vi "ErrorHandlerModularLoop vxm.vi"(8 "error in (no error)":errorcluster, 9 "exit event source":refnum<user-event>, 11 "MessageQues":T1) -> (0 "error out":errorcluster)   [LabVIEW 2019]
doc: "The Error hanlder Loop handles errors from all other Loops in the Multiple Loop Application Framework.\n\nThe DAQ Loop might need special handling, placeholde only now.\n\nMain and Analysis are set up to just Flush their ques, clear the error and pop open an OK dialog.\n***Not sure how we'll handle an error where messages are continually dropped on the Analysis/Main Que, causing the same error to repeat over and over - handle when needed."
uses:
  MessageQue/VXM Main Test App/MultipleMessageQues vxm.ctl
  MessageQue/MessageQue.ctl
  MessageQue/MessageCluster.ctl
  <vilib>/Utility/error.llb/DialogTypeEnum.ctl
  MessageQue/MessageQue.lvlib
  UserEvent-ExitEventLoop/UserEvent-ExitEventLoop.lvlib
panel:
  out "i":i32
  out "Command":string
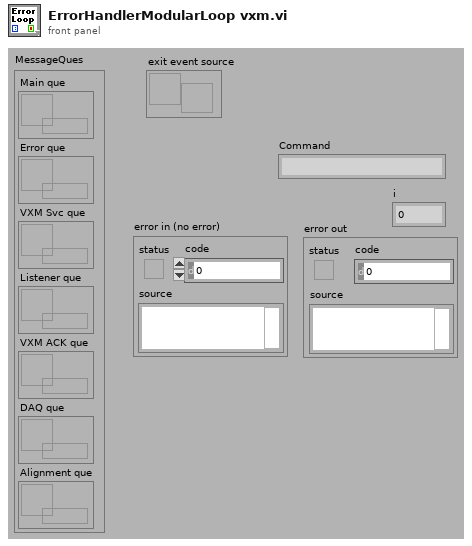
[diagram p1: front panel]
types:
  T1 = typedef "MultipleMessageQues vxm.ctl" = cluster{"Main que":T2, "Error que":T2, "VXM Svc que":T2, "Listener que":T2, "VXM ACK que":T2, "DAQ que":T2, "Alignment que":T2}
  T2 = typedef "MessageQue.lvlib/MessageQue.ctl" = refnum<queue>
  T3 = typedef "DialogTypeEnum.ctl" = enum16{"no dialog", "OK message", "continue or stop message", "auto error handling dialog", "OK message + warnings", "continue/stop + warnings"}
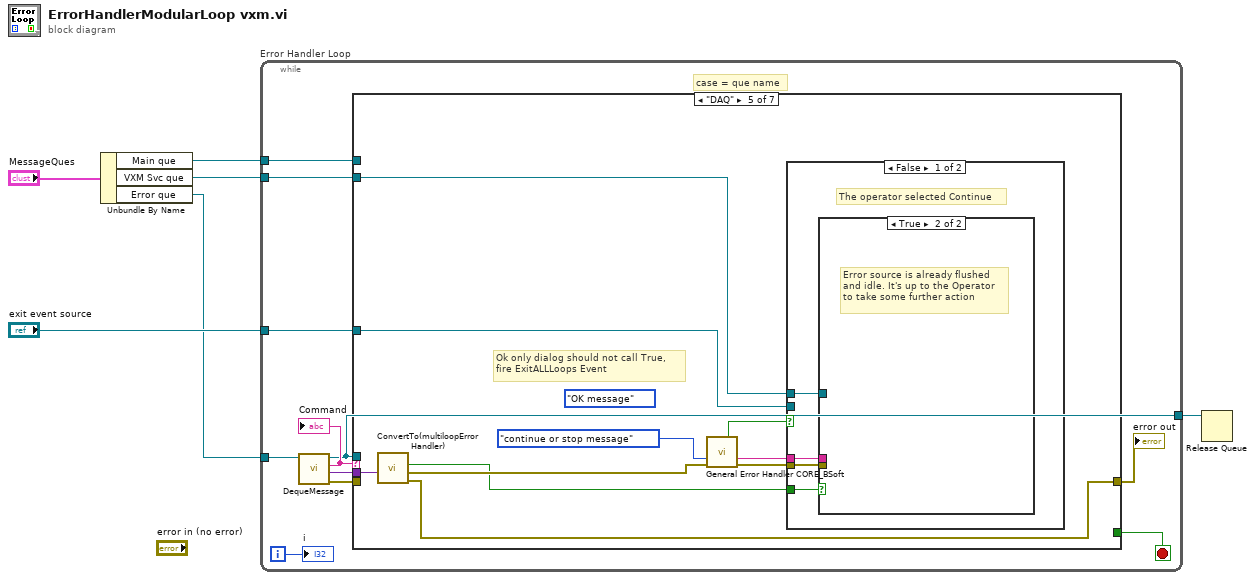
[diagram p0: block diagram]
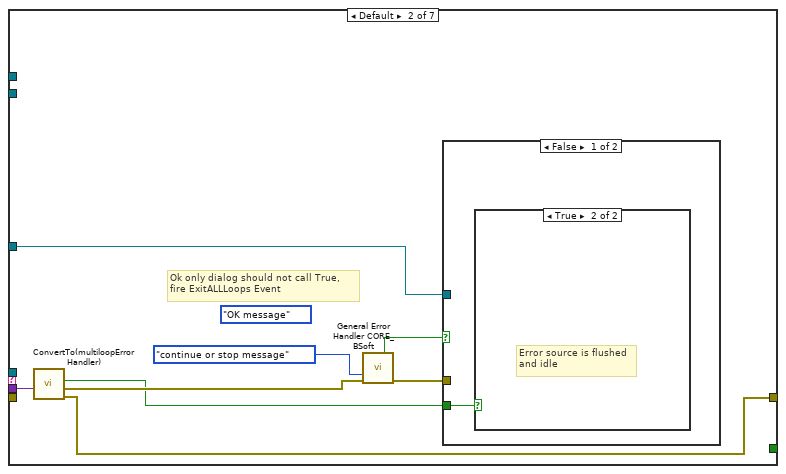
[diagram p3: hidden frame]
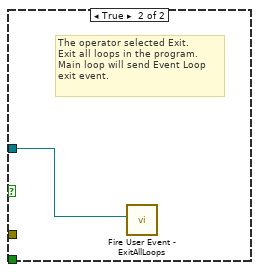
[diagram p5: hidden frame]
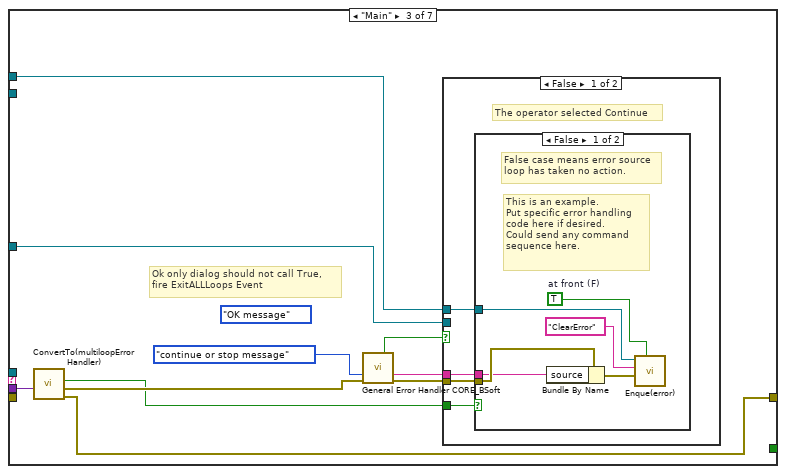
[diagram p6: hidden frame]
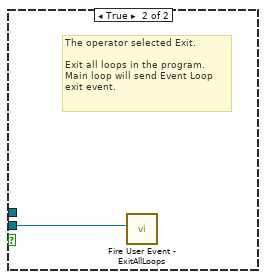
[diagram p8: hidden frame]
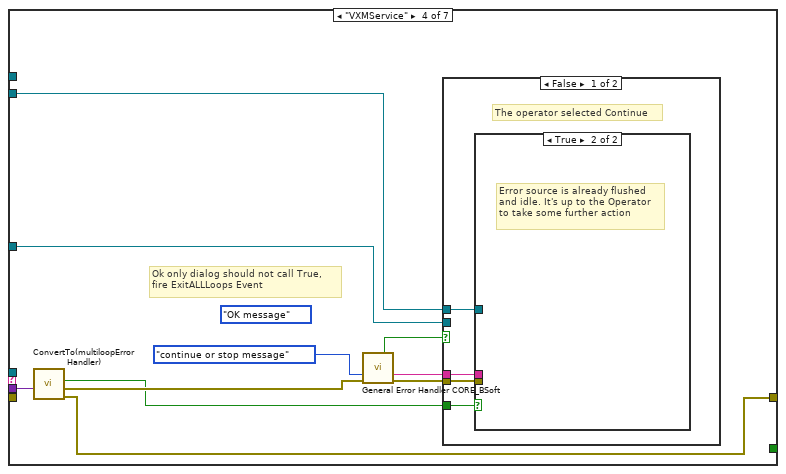
[diagram p9: hidden frame]
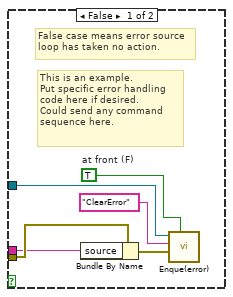
[diagram p10: hidden frame]
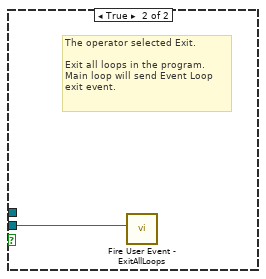
[diagram p11: hidden frame]
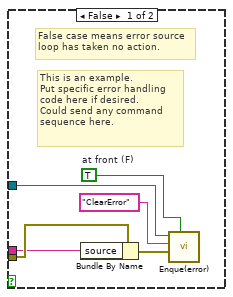
[diagram p12: hidden frame]
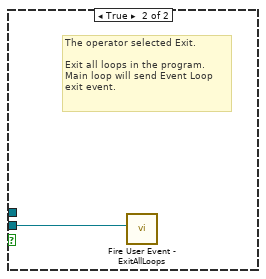
[diagram p13: hidden frame]
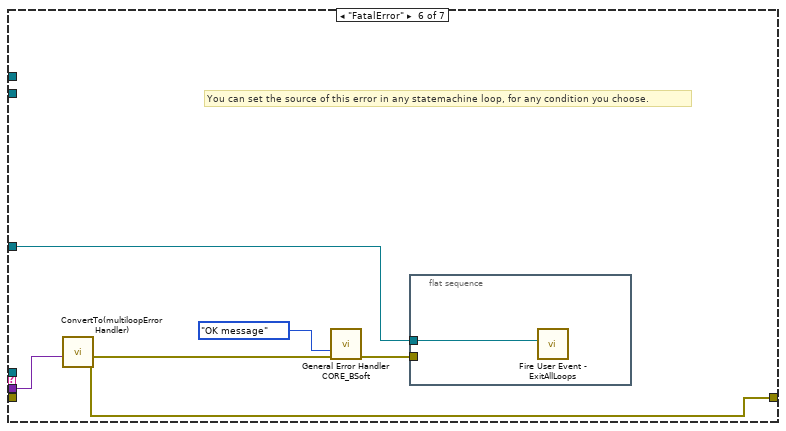
[diagram p14: hidden frame]
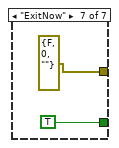
[diagram p15: hidden frame]
diagram:
  n1 = Unbundle By Name("MessageQues") -> ("Main que"=w3:T2, "VXM Svc que"=w4:T2, "Error que"=w2:T2)
  n2 = while "Error Handler Loop" {
    tunnel: w2 -> [w17]
    tunnel: w3 -> [w12]
    tunnel: w4 -> [w11]
    tunnel: "exit event source" -> [w9]
    tunnel: [w8] -> w5
    i -> [w16]
    stop <- w13 stop-if-true
    # "case = que name"
    n3 = call "DequeMessage.vi"("Message que"=w17) -> ("error out"=w14:errorcluster, "Message Payload"=w7:variant, "Message Command"=w15:string, "Message que out"=w8:T2)  [unwired: 5 in, 2 out]
    "Command" <- w15
    n4 = case shown="\"DAQ\"" w15 {
      tunnel: w8 -> [_ _ _ _ _ _ _]
      tunnel: [w18 w25 w37 w58 w79 w96 errorcluster {"status"=FALSE, "code"=0, "source"=""} ("error in (no error)")] -> w10
      tunnel: w14 -> [w18 _ _ _ _ _ _]
      tunnel: [_ _ _ _ _ _ TRUE] -> w13
      tunnel: w7 -> [_ w24 w36 w57 w78 w97 _]
      tunnel: w12 -> [_ _ w29 _ _ _ _]
      tunnel: w11 -> [_ _ _ w50 w71 _ _]
      tunnel: w9 -> [_ w26 w38 w59 w80 w92 _]
      frame "idle" {
      }
      frame Default {
        (unwired) DialogTypeEnum."OK message" ("type of dialog (OK msg:1)")
        # "Ok only dialog should not call True,\nfire ExitALLLoops Event"
        n5 = call "ConvertTo(multiloopErrorHandler).vi"("Message Payload"=w24) -> ("error out"=w25:errorcluster, "Message Payload error"=w20:errorcluster, "Handle Loop Que"=w19:bool)  [unwired: 8 in]
        n6 = call "General Error Handler CORE_BSoft.vi"("type of dialog (OK msg:1)"=DialogTypeEnum."continue or stop message", "error in (no error)"=w20) -> ("stop event propagated"=w23:bool, "error out"=w21:errorcluster)  [unwired: 8 in, 4 out]
        n7 = case shown="False" w23 {
          tunnel: w26 -> [_ w28]
          tunnel: w21 -> [_ _]
          tunnel: w19 -> [w27 _]
          frame False {
            n8 = case shown="True" w27 {
              frame False {
                # "False case means error source\nloop has taken no action."
                # "Default case can't send anything\nback to the source loop becasue\nit is the default and doesn't know\nwhich loop it is"
              }
              frame True {
                # "Error source is flushed\nand idle"
              }
            }
          }
          frame True {
            # "The operator selected Exit.\nExit all loops in the program.\nMain loop will send Event Loop\nexit event."
            n9 = call "Fire User Event - ExitAllLoops.vi"("user event ExitEventLoop"=w28) -> ()  [unwired: 10 in, 1 out]
          }
        }
      }
      frame "Main" {
        (unwired) DialogTypeEnum."OK message" ("type of dialog (OK msg:1)")
        # "Ok only dialog should not call True,\nfire ExitALLLoops Event"
        n10 = call "ConvertTo(multiloopErrorHandler).vi"("Message Payload"=w36) -> ("error out"=w37:errorcluster, "Message Payload error"=w32:errorcluster, "Handle Loop Que"=w31:bool)  [unwired: 8 in]
        n11 = call "General Error Handler CORE_BSoft.vi"("type of dialog (OK msg:1)"=DialogTypeEnum."continue or stop message", "error in (no error)"=w32) -> ("stop event propagated"=w35:bool, "message"=w30:string, "error out"=w33:errorcluster)  [unwired: 8 in, 3 out]
        n12 = case shown="False" w35 {
          tunnel: w38 -> [_ w49]
          tunnel: w33 -> [w41 _]
          tunnel: w31 -> [w42 _]
          tunnel: w30 -> [w40 _]
          tunnel: w29 -> [w39 _]
          frame False {
            # "The operator selected Continue"
            n13 = case shown="False" w42 {
              tunnel: w41 -> [w45 _]
              tunnel: w40 -> [w44 _]
              tunnel: w39 -> [w43 _]
              frame False {
                w46 = TRUE  # at front (F)
                # "False case means error source\nloop has taken no action."
                # "This is an example.\nPut specific error handling \ncode here if desired.\nCould send any command\nsequence here."
                n14 = Bundle By Name(cluster=w45, "source"=w44) -> (w47:errorcluster)
                n15 = call "Enque(error).vi"("at front (F)"=w46, "Message Payload  error cluster"=w47, "Message Command"="ClearError", "Message que"=w43) -> ()  [unwired: 6 in, 2 out]
              }
              frame True {
                # "Error source is already flushed\nand idle. It's up to the Operator\nto take some further action"
              }
            }
          }
          frame True {
            # "The operator selected Exit.\n\nExit all loops in the program.\nMain loop will send Event Loop\nexit event."
            n16 = call "Fire User Event - ExitAllLoops.vi"("user event ExitEventLoop"=w49) -> ()  [unwired: 10 in, 1 out]
          }
        }
      }
      frame "VXMService" {
        (unwired) DialogTypeEnum."OK message" ("type of dialog (OK msg:1)")
        # "Ok only dialog should not call True,\nfire ExitALLLoops Event"
        n17 = call "ConvertTo(multiloopErrorHandler).vi"("Message Payload"=w57) -> ("error out"=w58:errorcluster, "Message Payload error"=w53:errorcluster, "Handle Loop Que"=w52:bool)  [unwired: 8 in]
        n18 = call "General Error Handler CORE_BSoft.vi"("type of dialog (OK msg:1)"=DialogTypeEnum."continue or stop message", "error in (no error)"=w53) -> ("stop event propagated"=w56:bool, "message"=w51:string, "error out"=w54:errorcluster)  [unwired: 8 in, 3 out]
        n19 = case shown="False" w56 {
          tunnel: w59 -> [_ w70]
          tunnel: w54 -> [w62 _]
          tunnel: w52 -> [w63 _]
          tunnel: w51 -> [w61 _]
          tunnel: w50 -> [w60 _]
          frame False {
            # "The operator selected Continue"
            n20 = case shown="True" w63 {
              tunnel: w62 -> [w66 _]
              tunnel: w61 -> [w65 _]
              tunnel: w60 -> [w64 _]
              frame False {
                w67 = TRUE  # at front (F)
                # "False case means error source\nloop has taken no action."
                # "This is an example.\nPut specific error handling \ncode here if desired.\nCould send any command\nsequence here."
                n21 = Bundle By Name(cluster=w66, "source"=w65) -> (w68:errorcluster)
                n22 = call "Enque(error).vi"("at front (F)"=w67, "Message Payload  error cluster"=w68, "Message Command"="ClearError", "Message que"=w64) -> ()  [unwired: 6 in, 2 out]
              }
              frame True {
                # "Error source is already flushed\nand idle. It's up to the Operator\nto take some further action"
              }
            }
          }
          frame True {
            # "The operator selected Exit.\n\nExit all loops in the program.\nMain loop will send Event Loop\nexit event."
            n23 = call "Fire User Event - ExitAllLoops.vi"("user event ExitEventLoop"=w70) -> ()  [unwired: 10 in, 1 out]
          }
        }
      }
      frame "DAQ" {
        (unwired) DialogTypeEnum."OK message" ("type of dialog (OK msg:1)")
        # "Ok only dialog should not call True,\nfire ExitALLLoops Event"
        n24 = call "ConvertTo(multiloopErrorHandler).vi"("Message Payload"=w78) -> ("error out"=w79:errorcluster, "Message Payload error"=w74:errorcluster, "Handle Loop Que"=w73:bool)  [unwired: 8 in]
        n25 = call "General Error Handler CORE_BSoft.vi"("type of dialog (OK msg:1)"=DialogTypeEnum."continue or stop message", "error in (no error)"=w74) -> ("stop event propagated"=w77:bool, "message"=w72:string, "error out"=w75:errorcluster)  [unwired: 8 in, 3 out]
        n26 = case shown="False" w77 {
          tunnel: w80 -> [_ w91]
          tunnel: w75 -> [w83 _]
          tunnel: w73 -> [w84 _]
          tunnel: w72 -> [w82 _]
          tunnel: w71 -> [w81 _]
          frame False {
            # "The operator selected Continue"
            n27 = case shown="True" w84 {
              tunnel: w83 -> [w87 _]
              tunnel: w82 -> [w86 _]
              tunnel: w81 -> [w85 _]
              frame False {
                w88 = TRUE  # at front (F)
                # "False case means error source\nloop has taken no action."
                # "This is an example.\nPut specific error handling \ncode here if desired.\nCould send any command\nsequence here."
                n28 = Bundle By Name(cluster=w87, "source"=w86) -> (w89:errorcluster)
                n29 = call "Enque(error).vi"("at front (F)"=w88, "Message Payload  error cluster"=w89, "Message Command"="ClearError", "Message que"=w85) -> ()  [unwired: 6 in, 2 out]
              }
              frame True {
                # "Error source is already flushed\nand idle. It's up to the Operator\nto take some further action"
              }
            }
          }
          frame True {
            # "The operator selected Exit.\n\nExit all loops in the program.\nMain loop will send Event Loop\nexit event."
            n30 = call "Fire User Event - ExitAllLoops.vi"("user event ExitEventLoop"=w91) -> ()  [unwired: 10 in, 1 out]
          }
        }
      }
      frame "FatalError" {
        # "You can set the source of this error in any statemachine loop, for any condition you choose."
        n31 = call "ConvertTo(multiloopErrorHandler).vi"("Message Payload"=w97) -> ("error out"=w96:errorcluster, "Message Payload error"=w95:errorcluster)  [unwired: 8 in, 1 out]
        n32 = call "General Error Handler CORE_BSoft.vi"("type of dialog (OK msg:1)"=DialogTypeEnum."OK message", "error in (no error)"=w95) -> ("error out"=w94:errorcluster)  [unwired: 8 in, 5 out]
        n33 = flat-sequence {
          tunnel: w94 -> [_]
          tunnel: w92 -> [w98]
          frame #0 {
            n34 = call "Fire User Event - ExitAllLoops.vi"("user event ExitEventLoop"=w98) -> ()  [unwired: 10 in, 1 out]
          }
        }
      }
      frame "ExitNow" {
      }
    }
    "error out" <- w10
    "i" <- w16
  }
  n35 = Release Queue(queue=w5) -> ()  [unwired: 2 in, 3 out]
